vi "Get Pot Angle.vi"(1 "refnum name":string="My AnalogChannel RefNum") -> (0 "Angle":dbl)   [LabVIEW 2016]
doc: "DEPRECATED.\nGet the angle from a potentiometer.\nThis VI uses consts that are probaby coupled to a specific potentiometer tested, and now there's an official library that does the same thing."
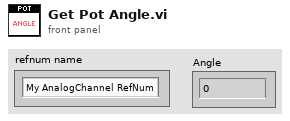
[diagram p1: front panel]
types:
  T1 = typedef "WPI_AnalogChannelDevRef.ctl" = cluster{"DevStatus":errorcluster, "Analog Channel":T2}
  T2 = typedef "FPGA_AIChannel.ctl" = enum8{"AI 0", "AI 1", "AI 2", "AI 3", "AI MXP 0", "AI MXP 1", "AI MXP 2", "AI MXP 3", "Invalid"}
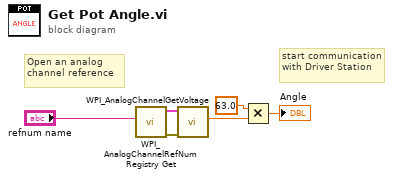
[diagram p0: block diagram]
diagram:
  # "start communication with Driver Station"
  # "Open an analog channel reference"
  n1 = call <vilib>:"WPI_AnalogChannelRefNum Registry Get.vi"("refnum name"="refnum name") -> ("error out"=w2:errorcluster, "AIDeviceRef"=w3:T1)  [unwired: 9 in]
  n2 = call <vilib>:"WPI_AnalogChannelGetVoltage.vi"("error in (no error)"=w2, "AIDeviceRef"=w3) -> ("Voltage"=w5:dbl)  [unwired: 9 out]
  n3 = Multiply(x=63.0, y=w5) -> (x*y=→"Angle":dbl)
